vi "LVObject to JSON - False - Pretty Print Disabled.vi"() -> ()   [LabVIEW 2017, in "Tests.lvlib" / "Pretty Print.lvlib"]
uses:
  Pretty Print.lvlib
  Flatten To JSON Object/Flatten To JSON Object.lvclass
  <vilib>/addons/_JKI Toolkits/Caraya/classes/Assert/Assert Equal Value_Variant.vi
  <vilib>/addons/_JKI Toolkits/Caraya/classes/Test/Test.lvclass
  <vilib>/addons/_JKI Toolkits/Caraya/classes/Assert/Assert.lvclass
  Temperature Forecast/Temperature Forecast.lvclass
panel:
  out "error out":errorcluster
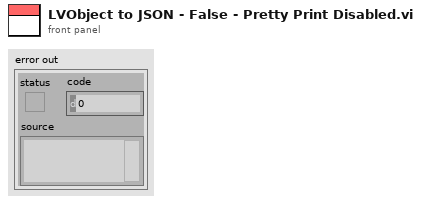
[diagram p1: front panel]
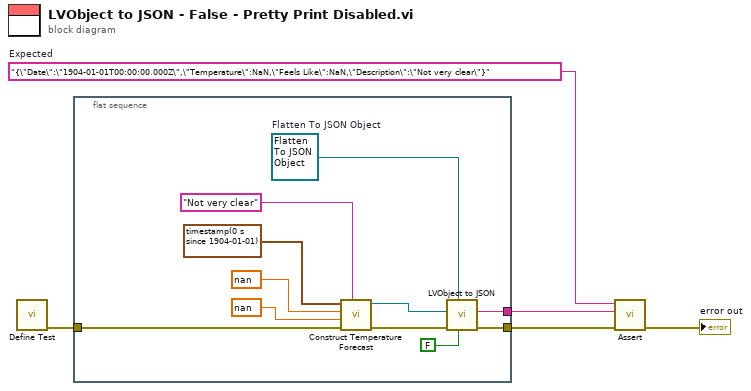
[diagram p0: block diagram]
diagram:
  w1 = "{\"Date\":\"1904-01-01T00:00:00.000Z\",\"Temperature\":NaN,\"Feels Like\":NaN,\"Description\":\"Not very clear\"}"  # Expected
  n1 = call <vilib>:"Define Test.vi"() -> ("error out"=w4:errorcluster)  [unwired: 11 in]
  n2 = flat-sequence {
    tunnel: w4 -> [w9]
    tunnel: [w15] -> w3
    tunnel: [w14] -> w2
    frame #0 {
      w16 = refnum<class "Flatten To JSON Object.lvclass"> refnum  # Flatten To JSON Object
      n3 = call "Construct Temperature Forecast.vi"("Description"="Not very clear", "error in (no error)"=w9, "Feels Like [°C]"=nan, "Temperature [°C]"=nan, "Date"=timestamp(0 s since 1904-01-01)) -> ("error out"=w8:errorcluster, "Temperature Forecast"=w7:refnum<class "Temperature Forecast.lvclass">)  [unwired: 5 in]
      n4 = call-dynamic "LVObject to JSON.vi"("Pretty Print?"=FALSE, "LVClass Serializer"=w16, "error in (no error)"=w8, "Object"=w7) -> ("error out"=w15:errorcluster, "<JSON>Object"=w14:string)  [unwired: 6 in]
    }
  }
  n5 = call-poly <vilib>:"Assert.vi"("error in (no error)"=w3, "Y"=w2, "X"=w1) -> ("error out"=→"error out":errorcluster)  [unwired: 8 in]
